vi "Auto_Drive_Test.vi"(8 "Timer?":bool, 9 "Duration":u32=3500, 10 "distance":dbl=88.0 format="%#_13g", 11 "Drive Effort":dbl=1000.0) -> ()   [LabVIEW 2016]
uses:
  <vilib>/Rock Robotics/WPI/SafetyOutput/WPI_SafetyOutputConfigMenu.ctl
panel:
  in  "Max Error":dbl=100.0 format="%#_13g"
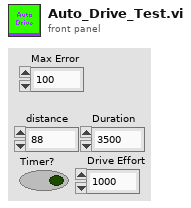
[diagram p1: front panel]
types:
  T1 = typedef "WPI_SafetyOutputConfigMenu.ctl" = enum16{"Enable", "Disable"}
  T2 = typedef "WPI_MotorControlDeviceRef.ctl" = cluster{"DeviceStatus":errorcluster, "Type":T3, "PWM":cluster{"PWM Channel":T4, "DeadBand":T5}, "CAN":cluster{"Device Number":u8, "SetOutput VI Ref":variant, "GetOutput VI Ref":variant, "Enable VI Ref":variant, "Disable VI Ref":variant, "Data":variant}, "Invert":bool}
  T3 = typedef "WPI_MotorControlType.ctl" = enum16{"PWM", "CAN"}
  T4 = typedef "FPGA_DIOPWMChannel.ctl" = enum8{"PWM 0", "PWM 1", "PWM 2", "PWM 3", "PWM 4", "PWM 5", "PWM 6", "PWM 7", "PWM 8", "PWM 9", "PWM MXP 0", "PWM MXP 1", "PWM MXP 2", "PWM MXP 3", "PWM MXP 4", "PWM MXP 5", "PWM MXP 6", "PWM MXP 7", "PWM MXP 8", "PWM MXP 9", "Invalid"}
  T5 = typedef "WPI_PWMDeadband.ctl" = cluster{"Name":string, "maxPositivePwm":i32, "minPositivePwm":i32, "centerPwm":i32, "maxNegativePwm":i32, "minNegativePwm":i32, "angularRange":u16}
  T6 = typedef "WPI_CANTalonSRX_GlobalStatus.ctl" = cluster{"Applied Throttle":dbl, "Module Enabled":bool, "CAN Error":errorcluster, "Closed Loop Error":dbl, "Forward Limit Switch Closed":bool, "Reverse Limit Switch Closed":bool, "Sensor Position":dbl, "Sensor Velocity":dbl, "Current":dbl, "Sticky Fault - Over Temp":bool, "Sticky Fault - Under Voltage":bool, "Sticky Fault - Forward Limit":bool, "Sticky Fault - Reverse Limit":bool, "Sticky Fault - Forward Soft Limit":bool, "Sticky Fault - Reverse Soft Limit":bool, "Brake is Enabled":bool, "Encoder Position":dbl, "Encoder Velocity":dbl, "Encoder Index Count":dbl, "Encoder A Pin State":bool, "Encoder B Pin State":bool, "Encoder Index Pin State":bool, "Analog In":dbl, "Analog In Velocity":dbl, "Temperature (C)":dbl, "Battery Voltage":dbl, "Control 5 Is Supported":bool, "Current Profile Slot Select":dbl, "Pos Div 8":bool, "Vel Div 4":bool, "Pulse Width Position":i32, "Pulse Width Velocity":i32, "Pulse Width Rise To Rise (us)":i32, "Pulse Width Rise To Fall (us)":i32, "Mot Prof Active Is Under Run":bool, "Mot Prof Active Has Under Run":bool, "Mot Prof Active Is Last":bool, "Mot Prof Active Velocity Only":bool, "Mot Prof Active Is Valid":bool, "Mot Prof Buffer Is Full":bool, "Mot Prof Active Profile Slot Select":i32, "Mot Prof NextID":i32, "Mot Prof Count":i32, "Mot Prof Active Velocity":dbl, "Mot Prof Active Position":dbl, "Mot Prof Output Enable":i32}
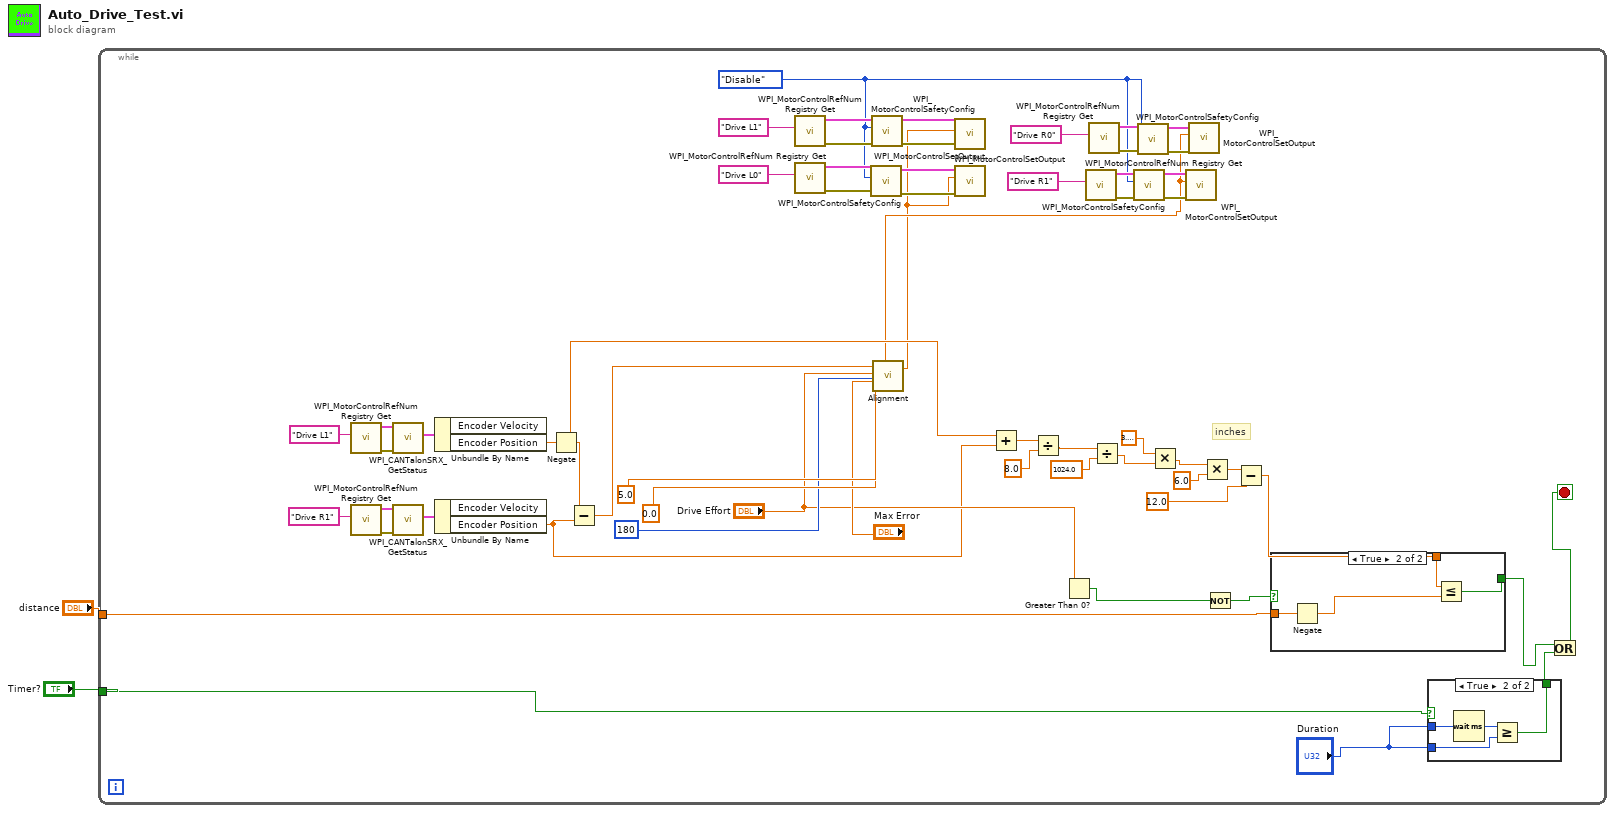
[diagram p0: block diagram]
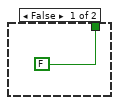
[diagram p2: hidden frame]
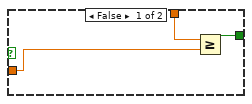
[diagram p3: hidden frame]
diagram:
  n1 = while {
    tunnel: "distance" -> [w42]
    tunnel: "Timer?" -> [w37]
    stop <- w32 stop-if-true
    w13 = WPI_SafetyOutputConfigMenu."Disable" ("mode")
    # "inches"
    n2 = call <vilib>:"WPI_MotorControlRefNum Registry Get.vi"("refnum name"="Drive L1") -> ("error out"=w54:errorcluster, "MotorControlDevRef"=w59:T2)  [unwired: 9 in]
    n3 = call <vilib>:"WPI_MotorControlRefNum Registry Get.vi"("refnum name"="Drive R1") -> ("error out"=w57:errorcluster, "MotorControlDevRef"=w58:T2)  [unwired: 9 in]
    n4 = call <vilib>:"WPI_CANTalonSRX_GetStatus.vi"("error in (no error)"=w54, "CAN Talon SRX Ref"=w59) -> ("Talon SRX Status"=w56:T6)  [unwired: 7 in, 2 out]
    n5 = call <vilib>:"WPI_CANTalonSRX_GetStatus.vi"("error in (no error)"=w57, "CAN Talon SRX Ref"=w58) -> ("Talon SRX Status"=w55:T6)  [unwired: 7 in, 2 out]
    n6 = Unbundle By Name(w56) -> ("Encoder Position"=w53:dbl)  [unwired: 1 out]
    n7 = Unbundle By Name(w55) -> ("Encoder Position"=w3:dbl)  [unwired: 1 out]
    n8 = Negate(x=w53) -> (-x=w12:dbl)
    n9 = Subtract(x=w12, y=w3) -> (x-y=w4:dbl)
    n10 = call <vilib>:"WPI_MotorControlRefNum Registry Get.vi"("refnum name"="Drive L1") -> ("error out"=w28:errorcluster, "MotorControlDevRef"=w29:T2)  [unwired: 9 in]
    n11 = call <vilib>:"WPI_MotorControlRefNum Registry Get.vi"("refnum name"="Drive L0") -> ("error out"=w24:errorcluster, "MotorControlDevRef"=w25:T2)  [unwired: 9 in]
    n12 = call <vilib>:"WPI_MotorControlSafetyConfig.vi"("error in (no error)"=w24, "mode"=w13, "MotorControlDevRef"=w25) -> ("error out"=w22:errorcluster, "MotorControlDevRef"=w23:T2)  [unwired: 7 in]
    n13 = call <vilib>:"WPI_MotorControlSafetyConfig.vi"("error in (no error)"=w28, "mode"=w13, "MotorControlDevRef"=w29) -> ("error out"=w26:errorcluster, "MotorControlDevRef"=w27:T2)  [unwired: 7 in]
    n14 = call "Alignment.vi"("Range"=5.0, "Camera Feedback"=w4, "Target"=0.0, "POV"=180, "Max Error"="Max Error", "Effort Addition"="Drive Effort") -> ("Right Motor"=w8:dbl, "Left Motor"=w7:dbl)  [unwired: 11 in, 1 out]
    n15 = call <vilib>:"WPI_MotorControlSetOutput.vi"("error in (no error)"=w26, "Output"=w7, "MotorControlDevRef"=w27) -> ()  [unwired: 6 in, 3 out]
    n16 = call <vilib>:"WPI_MotorControlSetOutput.vi"("error in (no error)"=w22, "Output"=w7, "MotorControlDevRef"=w23) -> ()  [unwired: 6 in, 3 out]
    n17 = Add(x=w12, y=w3) -> (x+y=w52:dbl)
    n18 = Divide(x=w52, y=8.0) -> (x/y=w50:dbl)
    n19 = Greater Than 0?(x="Drive Effort") -> (x > 0?=w38:bool)
    n20 = call <vilib>:"WPI_MotorControlRefNum Registry Get.vi"("refnum name"="Drive R1") -> ("error out"=w16:errorcluster, "MotorControlDevRef"=w17:T2)  [unwired: 9 in]
    n21 = call <vilib>:"WPI_MotorControlRefNum Registry Get.vi"("refnum name"="Drive R0") -> ("error out"=w20:errorcluster, "MotorControlDevRef"=w21:T2)  [unwired: 9 in]
    n22 = Divide(x=w50, y=1024.0) -> (x/y=w48:dbl)
    n23 = call <vilib>:"WPI_MotorControlSafetyConfig.vi"("error in (no error)"=w16, "mode"=w13, "MotorControlDevRef"=w17) -> ("error out"=w15:errorcluster, "MotorControlDevRef"=w14:T2)  [unwired: 7 in]
    n24 = call <vilib>:"WPI_MotorControlSafetyConfig.vi"("error in (no error)"=w20, "mode"=w13, "MotorControlDevRef"=w21) -> ("error out"=w19:errorcluster, "MotorControlDevRef"=w18:T2)  [unwired: 7 in]
    n25 = Multiply(x=3.141592653589793, y=w48) -> (x*y=w46:dbl)
    n26 = call <vilib>:"WPI_MotorControlSetOutput.vi"("error in (no error)"=w15, "Output"=w8, "MotorControlDevRef"=w14) -> ()  [unwired: 6 in, 3 out]
    n27 = call <vilib>:"WPI_MotorControlSetOutput.vi"("error in (no error)"=w19, "Output"=w8, "MotorControlDevRef"=w18) -> ()  [unwired: 6 in, 3 out]
    n28 = Multiply(x=w46, y=6.0) -> (x*y=w41:dbl)
    n29 = Not(x=w38) -> (.not. x?=w30:bool)
    n30 = Subtract(x=w41, y=12.0) -> (x-y=w39:dbl)
    n31 = case shown="True" w30 {
      tunnel: [w67 w73] -> w34
      tunnel: w42 -> [w68 w71]
      tunnel: w39 -> [w69 w70]
      frame False {
        n32 = Greater Or Equal?(x=w69, y=w68) -> (x >= y?=w67:bool)
      }
      frame True {
        n33 = Negate(x=w71) -> (-x=w72:dbl)
        n34 = Less Or Equal?(x=w70, y=w72) -> (x <= y?=w73:bool)
      }
    }
    n35 = case shown="True" w37 {
      tunnel: "Duration" -> [_ w65]
      tunnel: [FALSE w64] -> w33
      tunnel: "Duration" -> [_ w63]
      frame False {
      }
      frame True {
        n36 = Wait (ms)(milliseconds to wait=w63) -> (millisecond timer value=w66:u32)
        n37 = Greater Or Equal?(x=w66, y=w65) -> (x >= y?=w64:bool)
      }
    }
    n38 = Or(x=w34, y=w33) -> (x .or. y?=w32:bool)
  }
